vi "SmoothRandomNumberGenerator.vi"(8 "Max step size":dbl, 9 "Bottom range":dbl, 10 "Top range":dbl, 11 "Old val":dbl) -> (3 "New val":dbl)   [LabVIEW 2023]
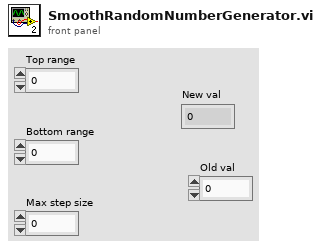
[diagram p1: front panel]
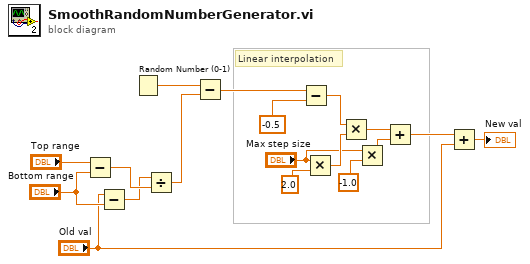
[diagram p0: block diagram]
diagram:
  # "Linear interpolation"
  n1 = Subtract(x="Top range", y="Bottom range") -> (x-y=w4:dbl)
  n2 = Subtract(x="Old val", y="Bottom range") -> (x-y=w3:dbl)
  n3 = Random Number (0-1)() -> (number: 0 to 1=w18:dbl)
  n4 = Divide(x=w3, y=w4) -> (x/y=w2:dbl)
  n5 = Subtract(x=w18, y=w2) -> (x-y=w16:dbl)
  n6 = Subtract(x=w16, y=-0.5) -> (x-y=w14:dbl)
  n7 = Multiply(x="Max step size", y=2.0) -> (x*y=w13:dbl)
  n8 = Multiply(x=w14, y=w13) -> (x*y=w12:dbl)
  n9 = Multiply(x="Max step size", y=-1.0) -> (x*y=w10:dbl)
  n10 = Add(x=w12, y=w10) -> (x+y=w1:dbl)
  n11 = Add(x=w1, y="Old val") -> (x+y=→"New val":dbl)
